vi "Configuration Process.vi"(8 "error in (no error)":errorcluster, 11 "View Model":T1) -> (0 "error out":errorcluster)   [LabVIEW 2017]
doc: "Configuration database process serves for Laod existing and save changed elevator time parameters"
uses:
  View Model/Controls/View Model.ctl
  Error Handler/Controls/Error Model.ctl
  Error Handler/Controls/Error EventData.ctl
  Error Handler/Controls/Error Type.ctl
  Elevator Controller/Controls/Elevator Model.ctl
  Elevator Controller/Controls/Elevator Overhead.ctl
  Elevator Controller/Controls/Elevator States.ctl
  Elevator Controller/Controls/Elevator Location.ctl
  Elevator Controller/Controls/Elevator Command Event.ctl
  Elevator Controller/Controls/Elevator Commands.ctl
  Controls/Configuration Model.ctl
  Controls/Configuration Data.ctl
  View Model/Controls/Shared Model.ctl
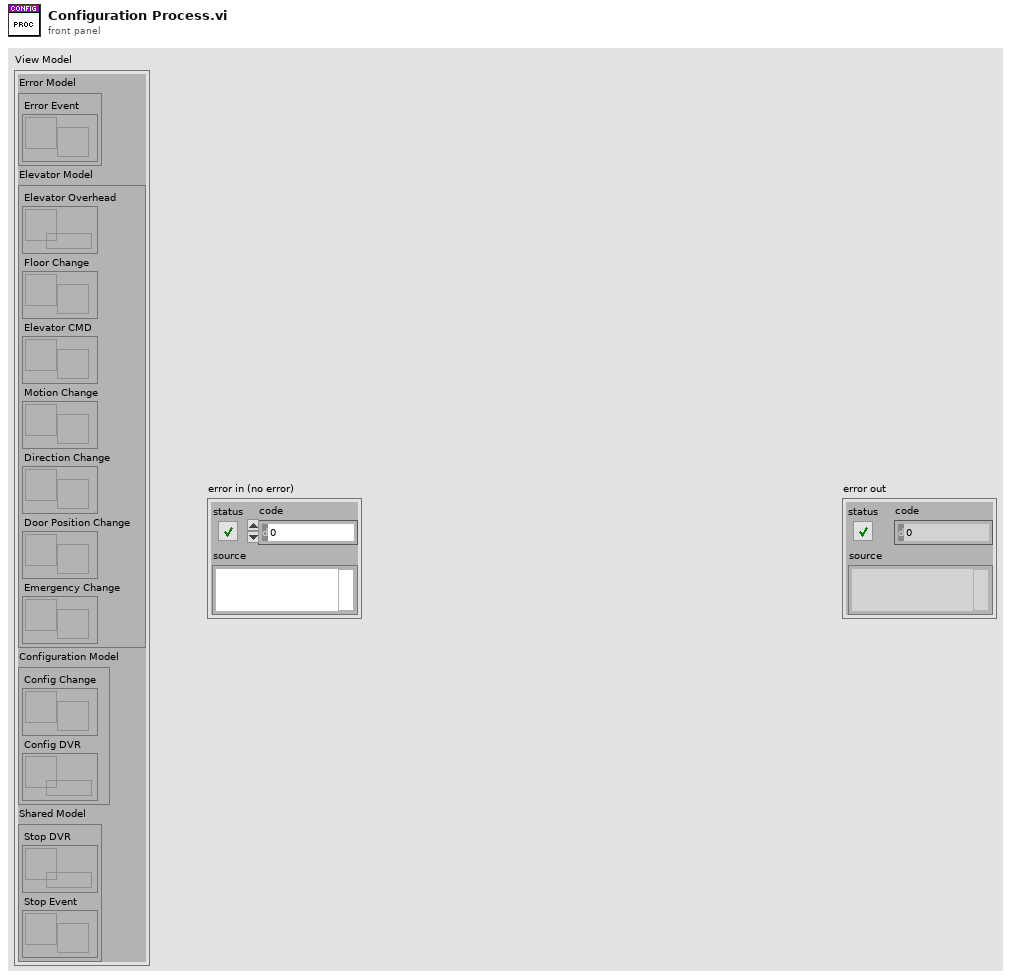
[diagram p1: front panel]
types:
  T1 = typedef "View Model.ctl" = cluster{"Error Model":T2, "Elevator Model":T3, "Configuration Model":T4, "Shared Model":T5}
  T2 = typedef "Error Model.ctl" = cluster{"Error Event":refnum<user-event>}
  T3 = typedef "Elevator Model.ctl" = cluster{"Elevator Overhead":refnum<data-value>, "Floor Change":refnum<user-event>, "Elevator CMD":refnum<user-event>, "Motion Change":refnum<user-event>, "Direction Change":refnum<user-event>, "Door Position Change":refnum<user-event>, "Emergency Change":refnum<user-event>}
  T4 = typedef "Configuration Model.ctl" = cluster{"Config Change":refnum<user-event>, "Config DVR":refnum<data-value>}
  T5 = typedef "Shared Model.ctl" = cluster{"Stop DVR":refnum<data-value>, "Stop Event":refnum<user-event>}
  T6 = typedef "Configuration Data.ctl" = cluster{"Door Open":dbl, "Door Close":dbl, "Travel Time":dbl, "Inactivity Time":dbl}
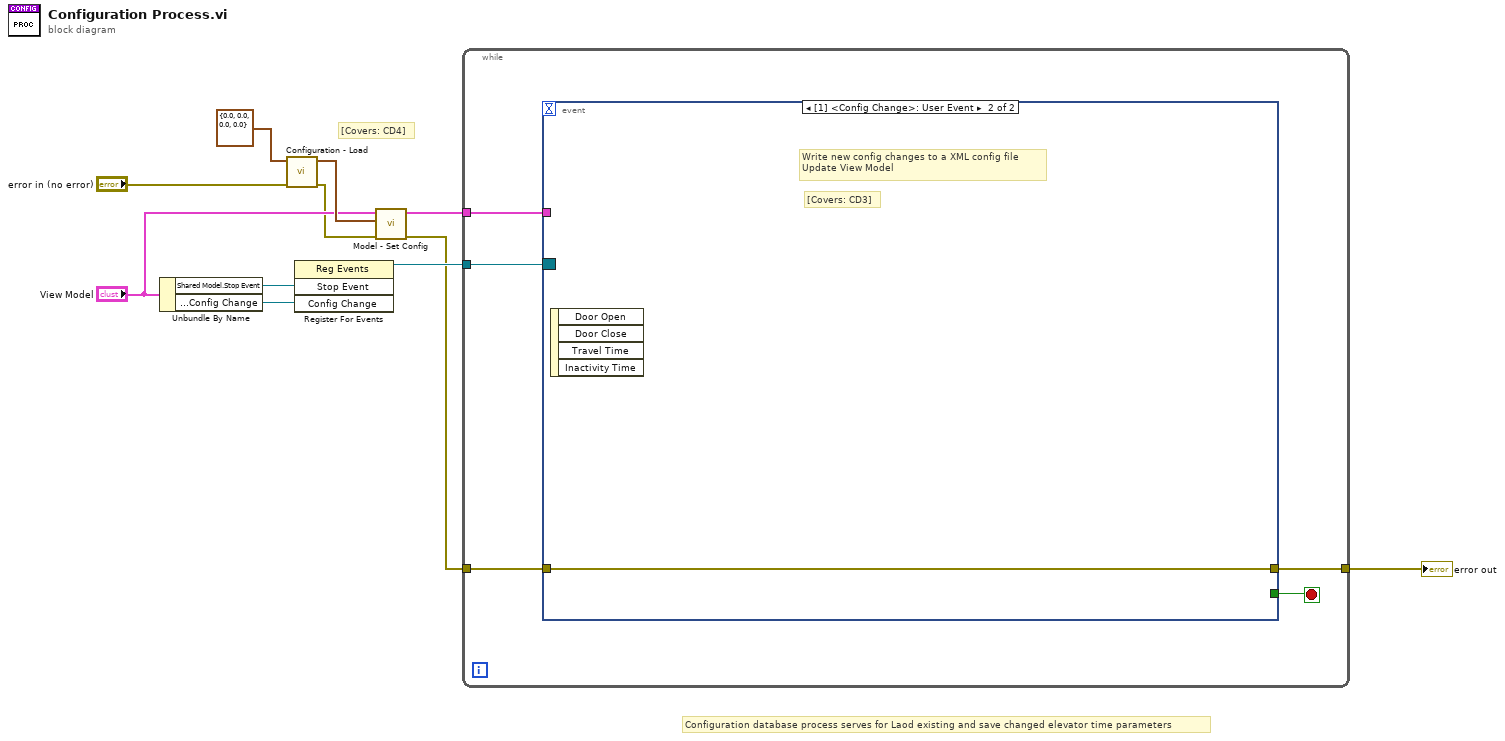
[diagram p0: block diagram]
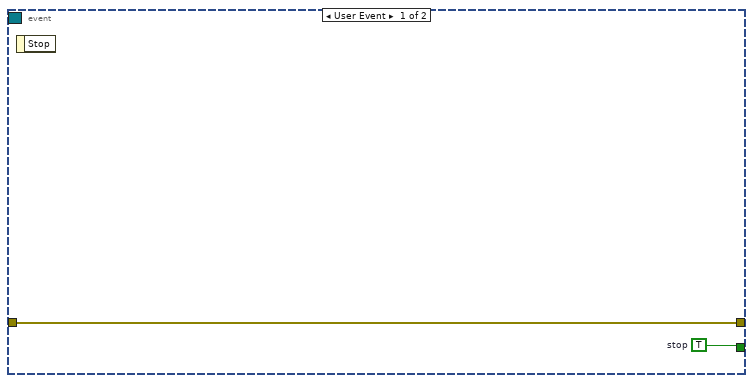
[diagram p2: hidden frame]
diagram:
  # "[Covers: CD4]"
  # "Configuration database process serves for Laod existing and save changed elevator time parameters"
  n1 = Unbundle By Name("View Model") -> ("Shared Model.Stop Event"=w11:refnum<user-event>, "Configuration Model.Config Change"=w10:refnum<user-event>)
  n2 = call "Configuration - Load.vi"("error in (no error)"="error in (no error)", "Configuration Data"=T6 {"Door Open"=0.0, "Door Close"=0.0, "Travel Time"=0.0, "Inactivity Time"=0.0}) -> ("error out"=w3:errorcluster, "Configuration Data"=w6:T6)  [unwired: 8 in]
  n3 = register-events(w11, w10) -> (reference out=w9:refnum<event-registration>)  [unwired: 2 in, 1 out]
  n4 = call "Model - Set Config.vi"("error in (no error)"=w3, "Configuration"=w6, "View Model"="View Model") -> ("error out"=w2:errorcluster, "View Model"=w1:T1)  [unwired: 7 in]
  n5 = while {
    tunnel: w9 -> [w16]
    tunnel: w2 -> [w15]
    tunnel: [w14] -> w8
    tunnel: w1 -> [w12]
    stop <- w13 stop-if-true
    n6 = event shown="[1] <Config Change>: User Event" {
      selector: w16 -> [_ _]
      dyn-events: _ -> [_ _]
      timeout: _ -> [_ _]
      tunnel: w15 -> [w18 w19]
      tunnel: [w18 w19] -> w14
      tunnel: [w17 _] -> w13
      tunnel: w12 -> [_ _]
      event User Event {
        w17 = TRUE  # stop
        n7 = event-data() -> ()  [unwired: 1 in, 1 out]
      }
      event User Event {
        # "[Covers: CD3]"
        # "Write new config changes to a XML config file\nUpdate View Model"
        n8 = event-data() -> ()  [unwired: 1 in, 4 out]
      }
    }
  }
  "error out" <- w8
